vi "frequency_sweep_agilent.vi"() -> ()   [LabVIEW 2017]
uses:
  controls/State.ctl
  controls/Data.ctl
  field_sweep_Agilent/Controls/Instruments.ctl
  <vilib>/Utility/error.llb/DialogType.ctl
  <vilib>/DAQmx/write.llb/DAQmx Write (Analog DBL 1Chan 1Samp).vi
  <vilib>/DAQmx/create/channels.llb/DAQmx Create Channel (AO-Voltage-Basic).vi
  <vilib>/DAQmx/miscellaneous.llb/DAQmx Fill In Error Info.vi
  <instrlib>/Keysight PNA Series/Keysight PNA Series.lvlib
panel:
  in  "Average Mode":i32(ring) items=["Point", "Sweep"]
  out "Field, Oe":dbl=17.9778 format="%#_4f"
  in  "IF Bandwidth":dbl(ring)=300.0 items=["10 Hz"=10.0, "30 Hz"=30.0, "100 Hz"=100.0, "300 Hz"=300.0, "1 KHz"=1000.0, "3 KHz"=3000.0, "10 KHz"=10000.0, "30 KHz"=30000.0]
  in  "Sweep Generation":i32(ring)=1 items=["Stepped", "Analog"]
  in  "Source Port":i32=1
  in  "Display Format":i32(ring) items=["Magnitude Linear", "Magnitude Logarithmic", "Phase", "Unwrapped phase", "Imaginary", "Real", "Polar", "Smith Chart", "Smith Admittance", "SWR", "Group Delay", "Kelvin", "Fahrenheit", "Celsius"]
  in  "S-parameter":i32(ring) items=["S11", "S12", "S21", "S22"]
  in  "Temp. Contr. Name (in)":refnum<visa-resource-name>="LakeShore336"
  in  "VNA name (in)":refnum<visa-resource-name>="vna"
  in  "Gaussmeter Name (in)":refnum<visa-resource-name>="Lakeshore_475"
  in  "DAQ channel (in)":tag="DAQ_6363/ao1"
  in  "Reference H Field On/Off":bool
  in  "Averaging Points":i32=1 min=1 max=3201 step=1
  in  "Exit Button":bool
  in  "Reference H Field (Oe)":dbl=4400.0 min=-4400.0 max=4400.0
  in  "H Field (Oe)":dbl=1000.0 min=-6000.0 max=6000.0
  in  "Save Button":bool
  out "Status":string="Off"
  out "Cursor":cluster{"x":dbl, "y":dbl} {"x" format="%.2f"; "y" format="%.5f"}
  out "Error Out":errorcluster={"status"=FALSE, "code"=1073676293, "source"="VISA Read in Keysight PNA Series.lvlib:Error Query.vi->Keysight PNA Series.lvlib:Close.vi->frequency_sweep_agilent.vi"}
  in  "Error In (no error)":errorcluster
  out "SpectrumGraph":cluster{"Field":dbl[], "Signal":dbl[]}(graph)
  in  "Start Button":bool
  in  "Stop Button":bool
  in  "Output Power (dBm)":dbl min=-25.0 max=50.0 step=0.5
  in  "Number of Points":i32=1000 min=1 max=3201 step=1
  in  "Stop frequency (GHz)":dbl=6.0 caption="Stop H Field (Oe)" min=0.01 max=26.5 format="%#_6f"
  in  "Start frequency (GHz)":dbl=1.0 min=0.01 max=26.5 format="%#_6f"
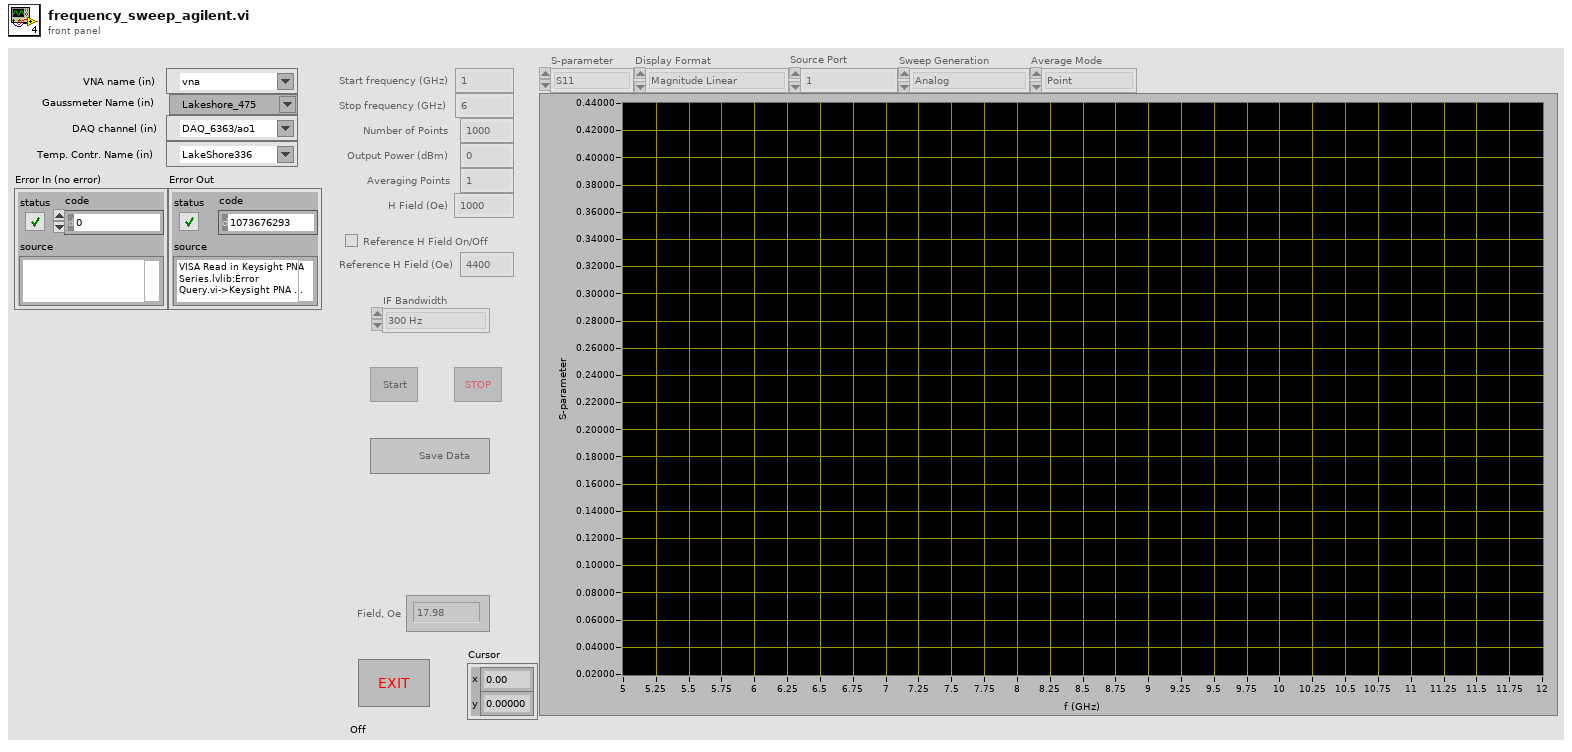
[diagram p1: front panel]
types:
  T1 = typedef "Instruments.ctl" = cluster{"Gaussmeter Name":refnum<visa-resource-name>, "VNA name":refnum<visa-resource-name>, "DAQ channel":tag, "DAQ task":refnum<k21>, "Temp. Contr. Name":refnum<visa-resource-name>}
  T2 = typedef "Data.ctl" = cluster{"Frequency":dbl[], "Signal":dbl[], "Ref signal":dbl[]}
  T3 = typedef "State.ctl" = enum16{"Init", "Idle", "Configuring", "Sweeping to ref", "Measuring ref", "Sweeping to H", "Measuring H", "Sweeping down", "Shutdown"}
  T4 = typedef "DialogType.ctl" = u16
  T5 = typedef "LVPoint32TypeDef.ctl" = cluster{"Horizontal":i32, "Vertical":i32}
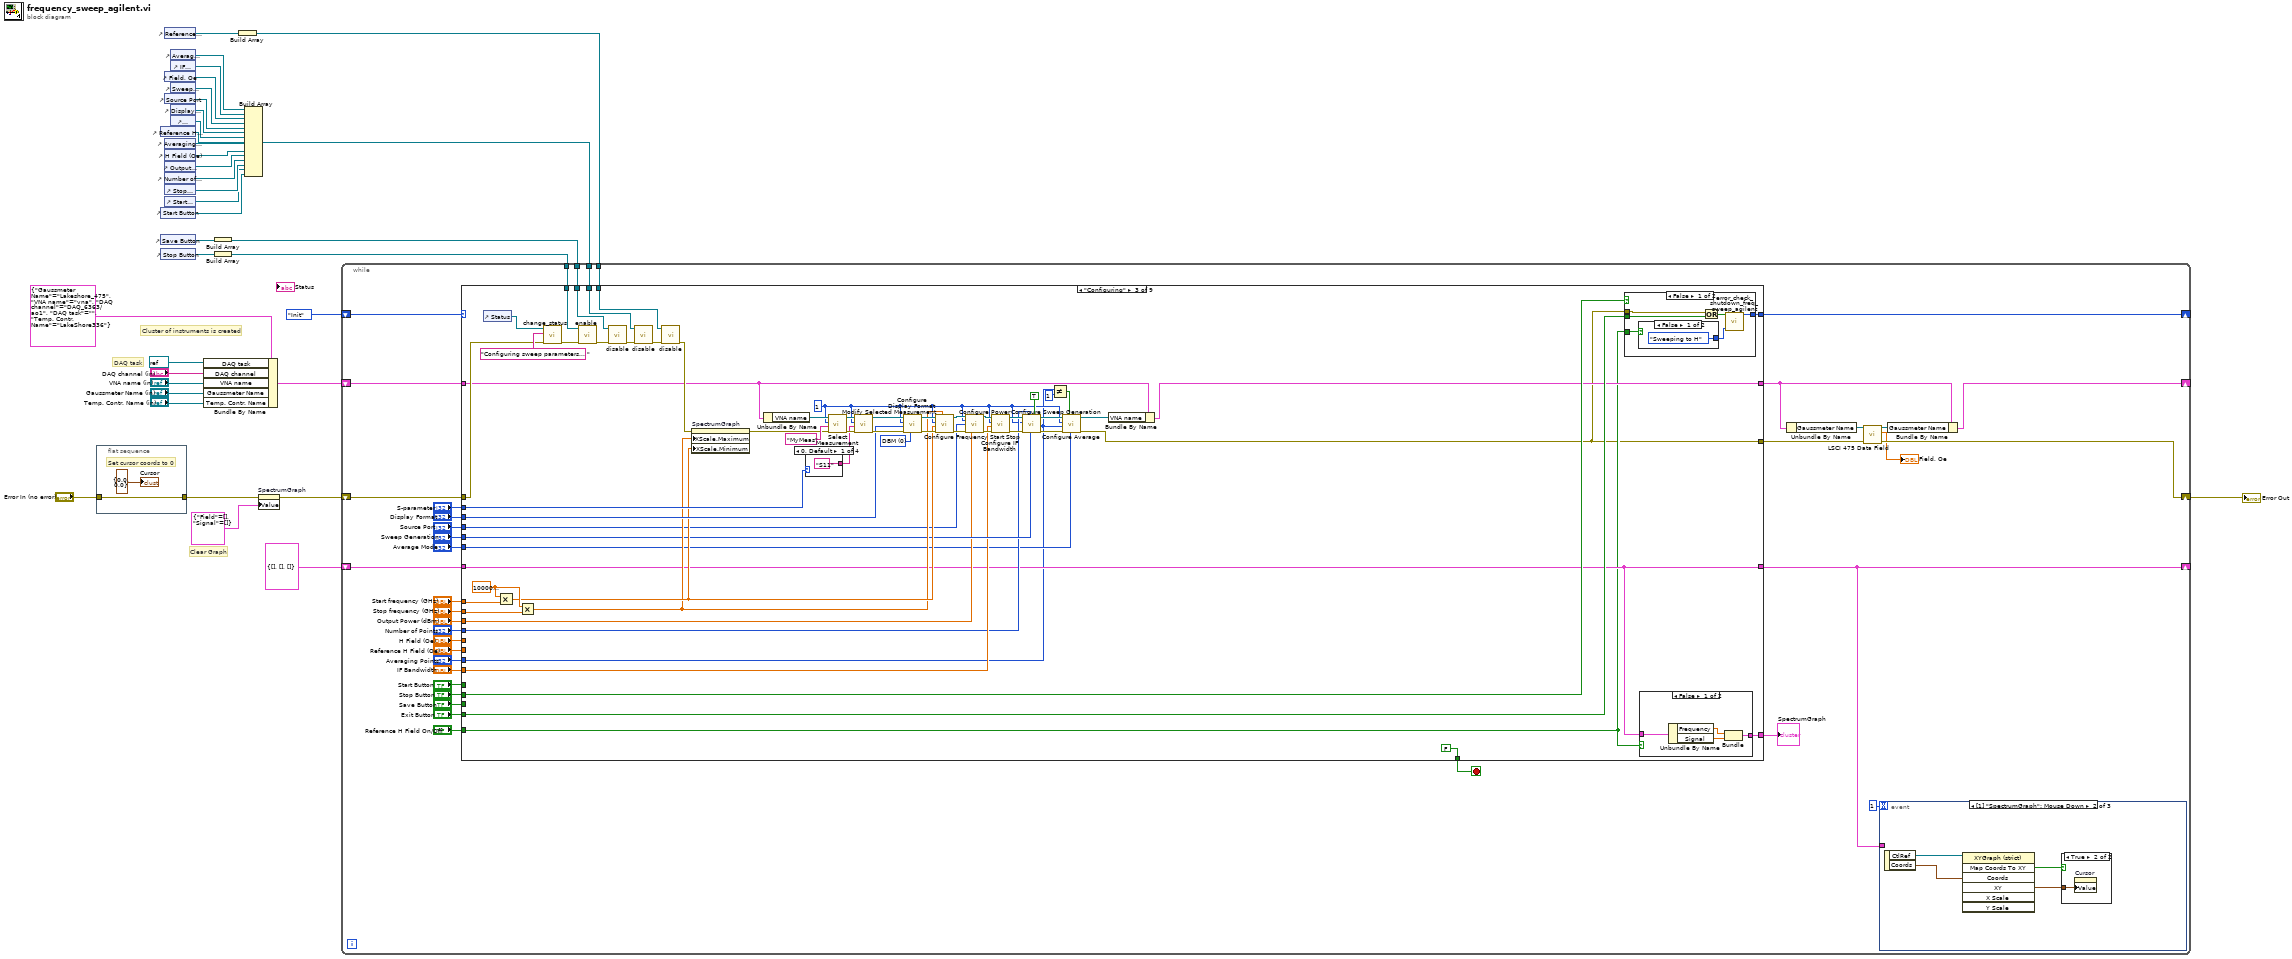
[diagram p0: block diagram]
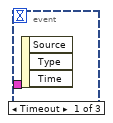
[diagram p2: hidden frame]
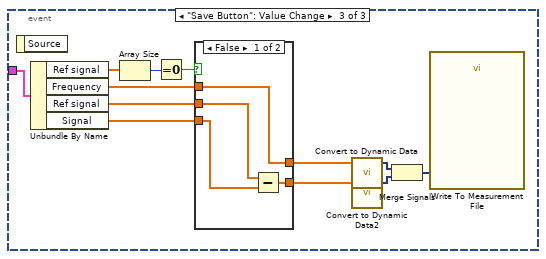
[diagram p4: hidden frame]
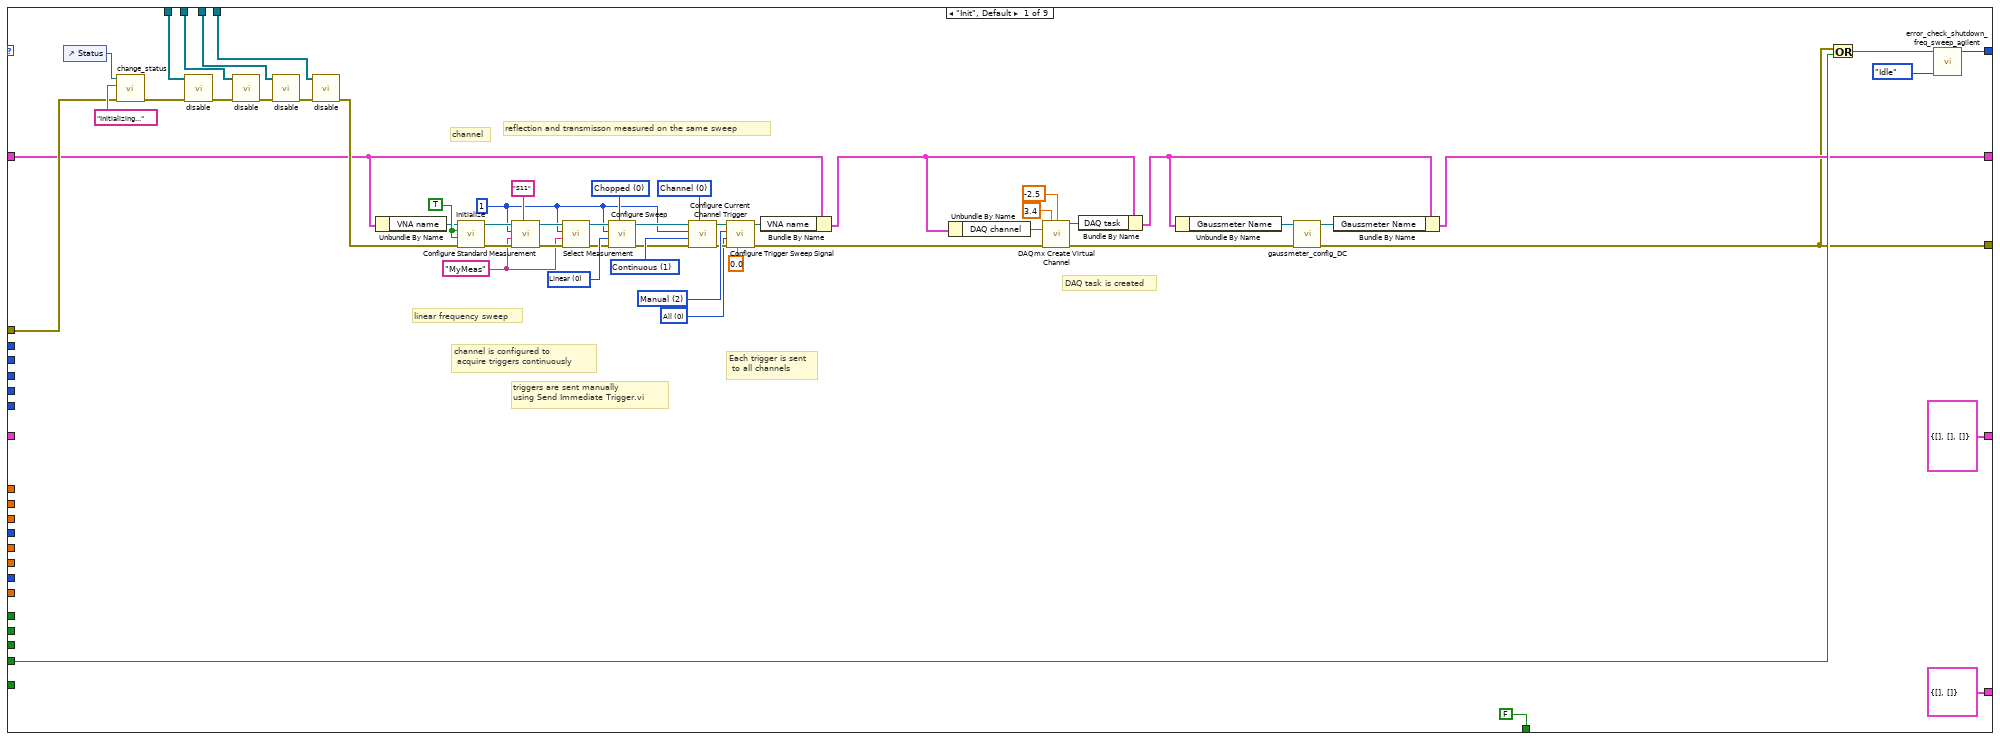
[diagram p6: hidden frame]
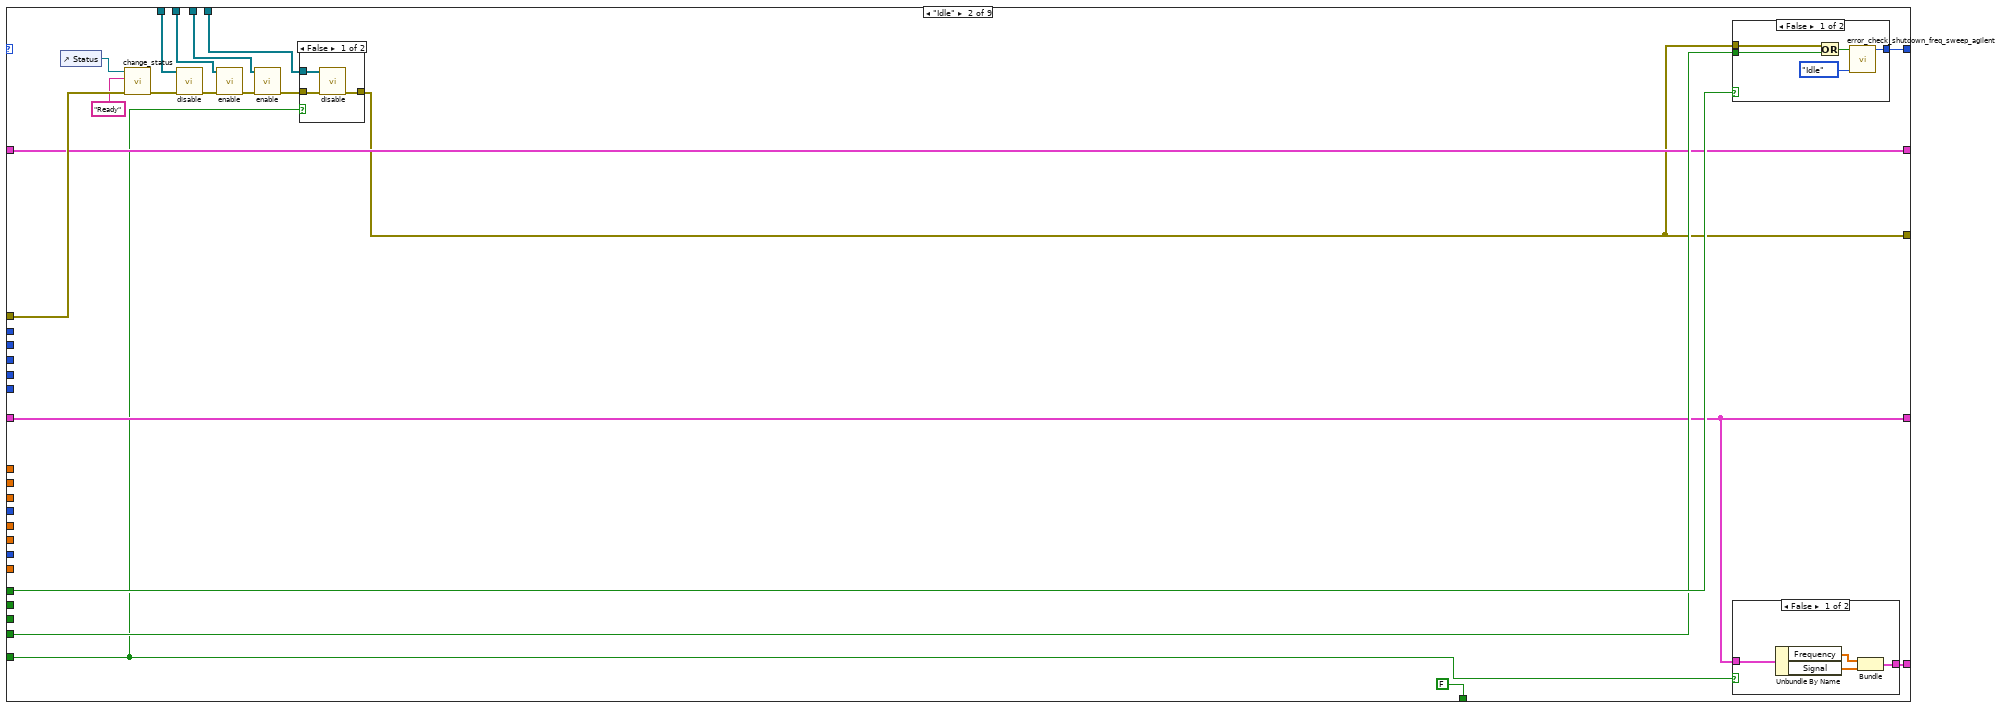
[diagram p7: hidden frame]
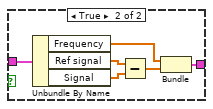
[diagram p8: hidden frame]
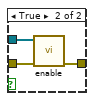
[diagram p9: hidden frame]
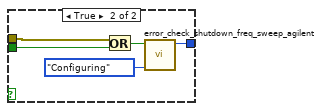
[diagram p10: hidden frame]
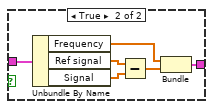
[diagram p11: hidden frame]
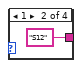
[diagram p12: hidden frame]
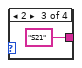
[diagram p13: hidden frame]
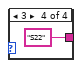
[diagram p14: hidden frame]
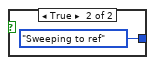
[diagram p15: hidden frame]
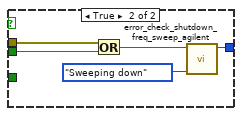
[diagram p16: hidden frame]
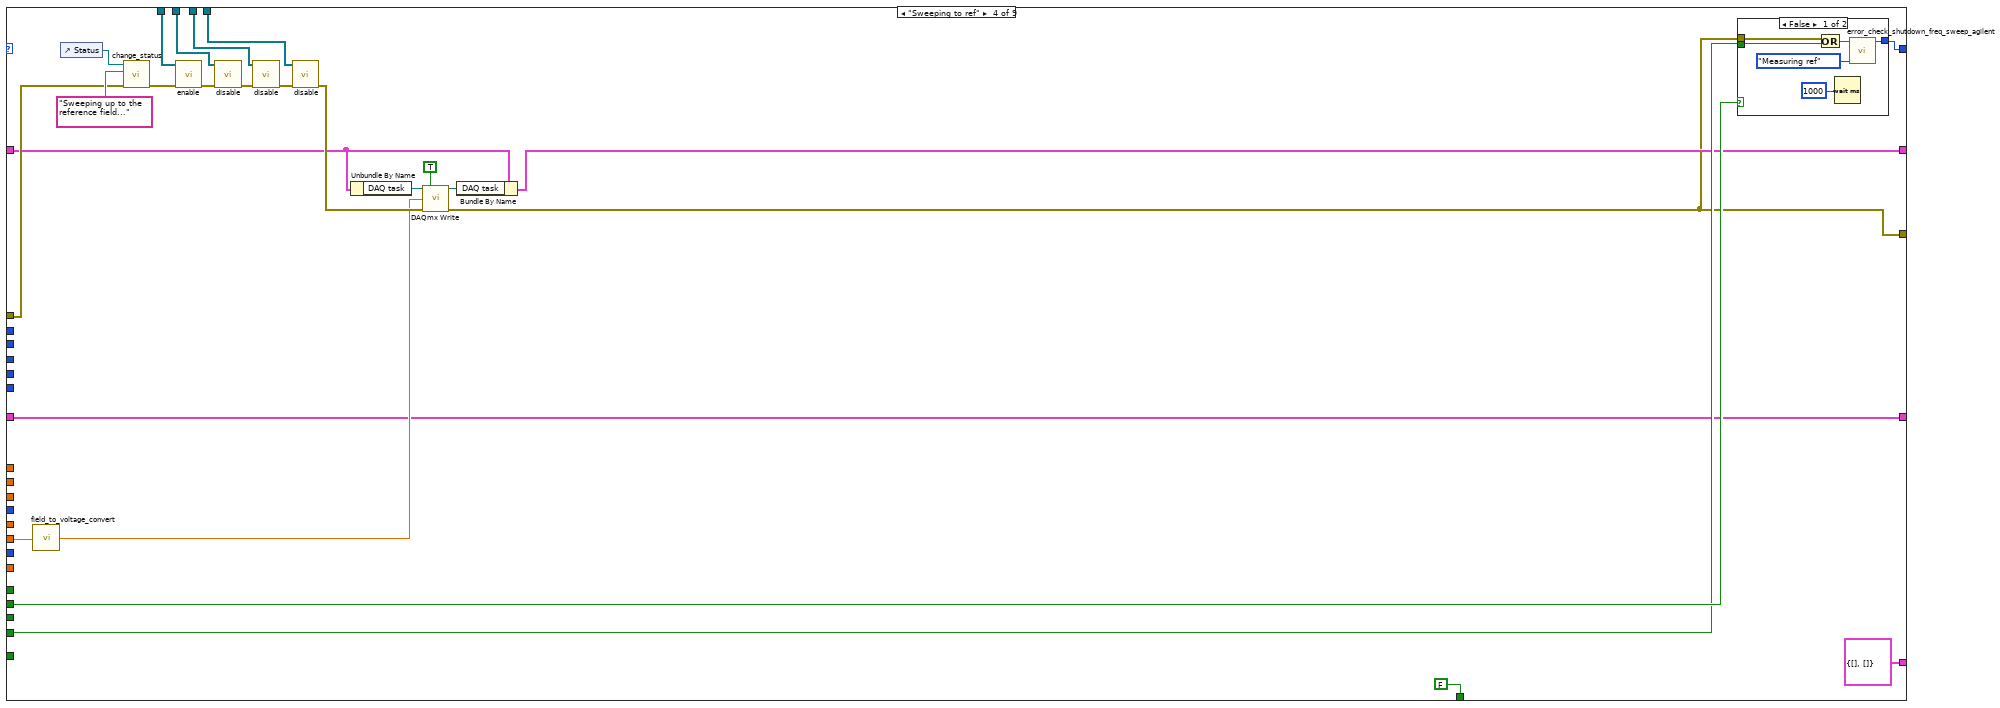
[diagram p17: hidden frame]
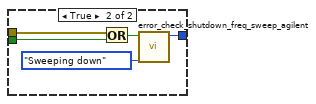
[diagram p18: hidden frame]
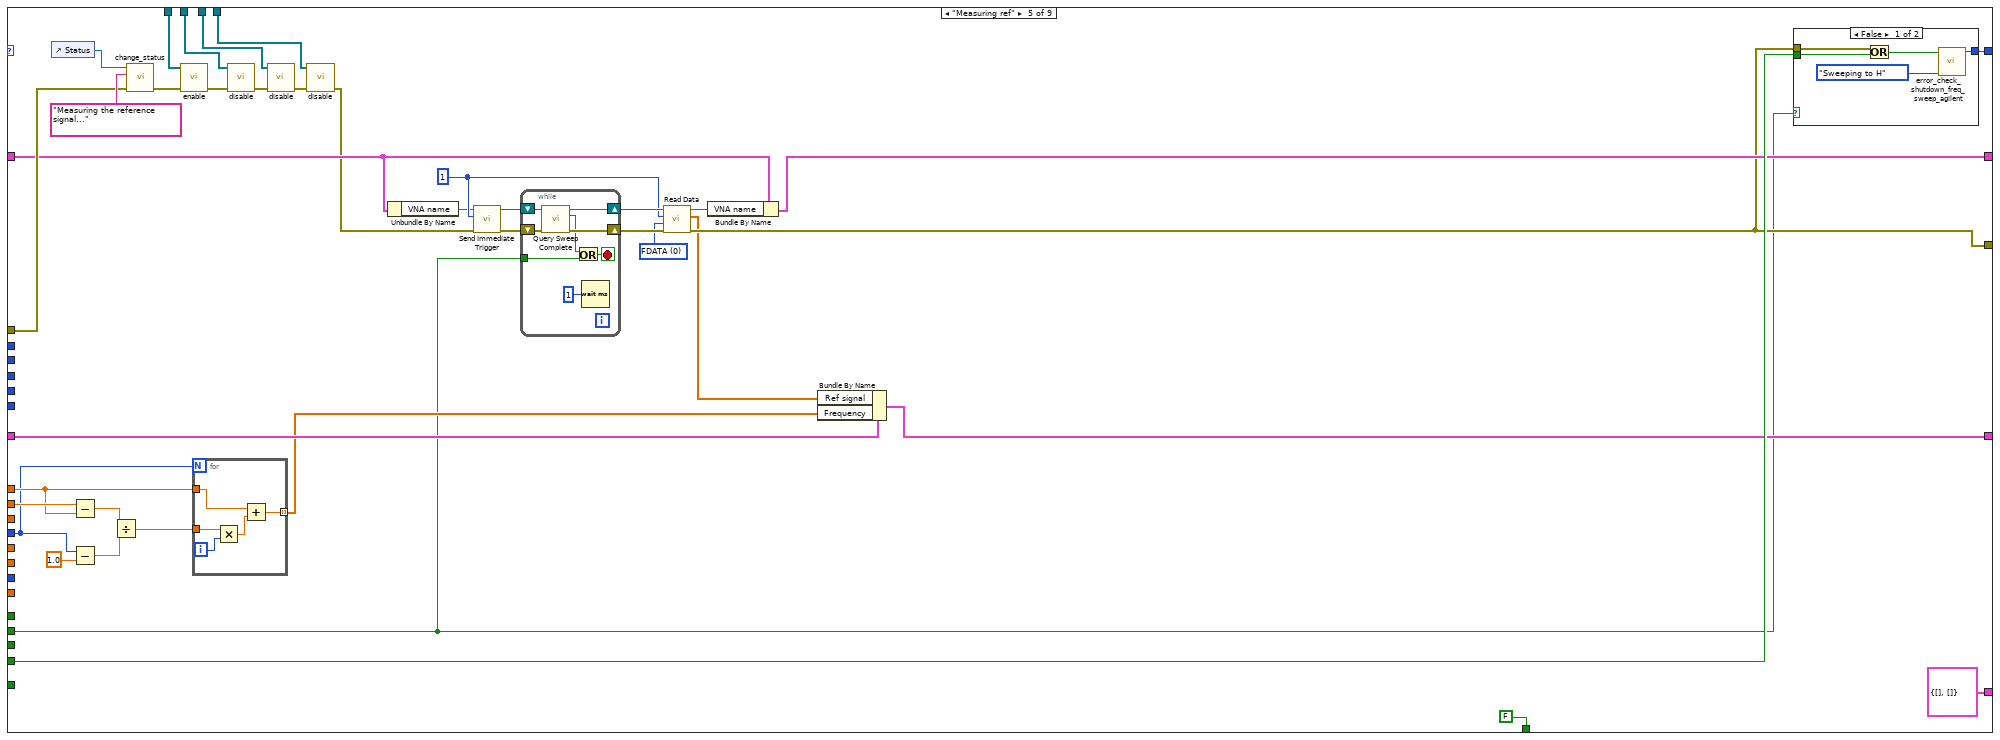
[diagram p19: hidden frame]
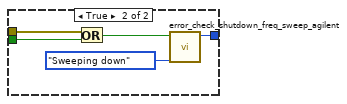
[diagram p20: hidden frame]
diagram:
  # "Cluster of instruments is created"
  # "DAQ task"
  # "Clear Graph"
  n1 = flat-sequence {
    tunnel: "Error In (no error)" -> [w38]
    tunnel: [w38] -> w9
    frame #0 {
      # "Set cursor coords to 0"
      "Cursor" <- cluster{"x":dbl, "y":dbl} {"x"=0.0, "y"=0.0} ("Cursor")
    }
  }
  n2 = control-ref of="Reference H Field On/Off"() -> (w8:refnum<vi>)
  n3 = control-ref of="Start Button"() -> (w18:refnum<vi>)
  n4 = control-ref of="Save Button"() -> (w28:refnum<vi>)
  n5 = control-ref of="Stop Button"() -> (w31:refnum<vi>)
  n6 = control-ref of="Reference H Field (Oe)"() -> (w20:refnum<vi>)
  n7 = control-ref of="Field, Oe"() -> (w3:refnum<vi>)
  n8 = control-ref of="Source Port"() -> (w5:refnum<vi>)
  n9 = control-ref of="Averaging Points"() -> (w26:refnum<vi>)
  n10 = control-ref of="H Field (Oe)"() -> (w36:refnum<vi>)
  n11 = control-ref of="Output Power (dBm)"() -> (w35:refnum<vi>)
  n12 = control-ref of="Number of Points"() -> (w34:refnum<vi>)
  n13 = control-ref of="Stop frequency (GHz)"() -> (w33:refnum<vi>)
  n14 = control-ref of="Start frequency (GHz)"() -> (w32:refnum<vi>)
  n15 = control-ref of="Average Mode"() -> (w1:refnum<vi>)
  n16 = control-ref of="IF Bandwidth"() -> (w2:refnum<vi>)
  n17 = control-ref of="Sweep Generation"() -> (w4:refnum<vi>)
  n18 = control-ref of="Display Format"() -> (w6:refnum<vi>)
  n19 = control-ref of="S-parameter"() -> (w7:refnum<vi>)
  n20 = Bundle By Name(cluster=T1 {"Gaussmeter Name"="Lakeshore_475", "VNA name"="vna", "DAQ channel"="DAQ_6363/ao1", "DAQ task"="", "Temp. Contr. Name"="LakeShore336"} ("Cluster"), "DAQ task"=refnum<k21> refnum ("task in"), "DAQ channel"="DAQ channel (in)", "VNA name"="VNA name (in)", "Gaussmeter Name"="Gaussmeter Name (in)", "Temp. Contr. Name"="Temp. Contr. Name (in)") -> (w11:T1)
  n21 = Build Array(w28) -> (w27:refnum<vi>[])
  n22 = Build Array(w31) -> (w29:refnum<vi>[])
  n23 = Build Array(w20) -> (w19:refnum<vi>[])
  n24 = Build Array(w1, w2, w3, w4, w5, w6, w7, w8, w26, w36, w35, w34, w33, w32, w18) -> (w30:refnum<vi>[])
  n25 = property on="SpectrumGraph" class="XYGraph (strict)"(error in=w9, "Value"=cluster{"Field":dbl[], "Signal":dbl[]} {"Field"=[], "Signal"=[]} ("SpectrumGraph")) -> (error out=w24:errorcluster)  [unwired: 1 in, 1 out]
  n26 = while {
    shift-right: [w57] -> _
    shift-left: State."Init" -> [w58]
    tunnel: w30 -> [w76]
    tunnel: w29 -> [w75]
    shift-right: [w44] -> w25
    shift-left: w24 -> [w74]
    tunnel: w27 -> [w73]
    shift-right: [w47] -> _
    shift-left: T2 {"Frequency"=[], "Signal"=[], "Ref signal"=[]} -> [w59]
    tunnel: w19 -> [w55]
    shift-right: [w41] -> _
    shift-left: w11 -> [w54]
    stop <- w68 stop-if-true
    n27 = case shown="\"Configuring\"" w58 {
      tunnel: w76 -> [w148 w172 w256 w308 w361 w408 w471 w527 w573]
      tunnel: w75 -> [w154 w174 w255 w310 w363 w411 w473 w525 w575]
      tunnel: w74 -> [w150 w169 w253 w306 w356 w406 w470 w528 w571]
      tunnel: [w145 w163 w248 w304 w354 w401 w450 w522 State."Shutdown" ("Enum")] -> w57
      tunnel: [w102 w158 w206 w290 w338 w390 w449 w503 w560] -> w46
      tunnel: w73 -> [w149 w173 w257 w309 w362 w409 w472 w526 w574]
      tunnel: "Start Button" -> [_ w166 _ _ _ _ _ _ _]
      tunnel: "Stop Button" -> [_ _ w250 w305 w325 w403 w435 _ _]
      tunnel: "Save Button" -> [_ _ _ _ _ _ _ _ _]
      tunnel: "Exit Button" -> [w146 w165 w249 w303 w355 w402 w468 w523 _]
      tunnel: [FALSE FALSE FALSE FALSE FALSE FALSE FALSE FALSE TRUE] -> w68
      tunnel: "Start frequency (GHz)" -> [_ _ w252 _ w332 _ w441 _ _]
      tunnel: "Stop frequency (GHz)" -> [_ _ w251 _ w333 _ w446 _ _]
      tunnel: "Output Power (dBm)" -> [_ _ w217 _ _ _ _ _ _]
      tunnel: "Number of Points" -> [_ _ w213 _ w331 _ w442 _ _]
      tunnel: "H Field (Oe)" -> [_ _ _ _ _ w404 _ _ _]
      tunnel: "Reference H Field (Oe)" -> [_ _ _ w301 _ _ _ _ _]
      tunnel: "Averaging Points" -> [_ _ w202 _ _ _ _ _ _]
      tunnel: w59 -> [_ w156 w211 w289 w330 w388 w448 w501 _]
      tunnel: [T2 {"Frequency"=[], "Signal"=[], "Ref signal"=[]} w156 w211 w289 w327 w388 w437 w501 T2 {"Frequency"=[], "Signal"=[], "Ref signal"=[]}] -> w47
      tunnel: "S-parameter" -> [_ _ w227 _ _ _ _ _ _]
      tunnel: "Reference H Field On/Off" -> [_ w155 w210 _ _ w387 w438 w500 _]
      tunnel: w55 -> [w139 w160 w244 w298 w350 w398 w465 w516 w565]
      tunnel: w54 -> [w114 w159 w215 w293 w341 w393 w454 w506 w544]
      tunnel: [w105 w159 w214 w292 w340 w392 w453 w504 w544] -> w42
      tunnel: "Display Format" -> [_ _ w226 _ _ _ _ _ _]
      tunnel: "Source Port" -> [_ _ w219 _ _ _ _ _ _]
      tunnel: "Sweep Generation" -> [_ _ w218 _ _ _ _ _ _]
      tunnel: "IF Bandwidth" -> [_ _ w216 _ _ _ _ _ _]
      tunnel: [cluster{"Frequency":dbl[], "Signal":dbl[]} {"Frequency"=[], "Signal"=[]} w157 w212 cluster{"Frequency":dbl[], "Signal":dbl[]} {"Frequency"=[], "Signal"=[]} cluster{"Frequency":dbl[], "Signal":dbl[]} {"Frequency"=[], "Signal"=[]} w389 w436 w502 cluster{"Frequency":dbl[], "Signal":dbl[]} {"Frequency"=[], "Signal"=[]}] -> w48
      tunnel: "Average Mode" -> [_ _ w205 _ _ _ _ _ _]
      frame "Init", Default {
        w121 = 0 items=["All", "Current"] ("Trigger Scope (0: All)")
        w122 = 0 items=["Channel", "Sweep", "Point", "Trace"] ("Trigger Mode (0: Channel)")
        w125 = 1 items=["Hold", "Continuous", "Groups", "Single"] ("Trigger Condition (1: Continuous)")
        w126 = 2 items=["Immediate", "External", "Manual"] ("Trigger Source (0: Immediate)")
        w132 = 0 items=["Chopped", "Alternate"] ("Sweep Mode (0: Chopped)")
        w133 = 0 items=["Linear", "Logarithmic", "Power", "CW", "Segment", "Phase"] ("Sweep Type (0: Linear)")
        w127 = "MyMeas" ("Measurement Name (CH1_S11_1)")
        w116 = 1 ("Channel (1)")
        w138 = TRUE ("ID Query (True)")
        # "DAQ task is created"
        # "channel"
        # "reflection and transmisson measured on the same sweep"
        # "Each trigger is sent\n to all channels"
        # "triggers are sent manually\nusing Send Immediate Trigger.vi"
        # "channel is configured to\n acquire triggers continuously"
        # "linear frequency sweep"
        n28 = control-ref of="Status"() -> (w152:refnum<vi>)
        n29 = call "change_status.vi"("error in (no error)"=w150, "String"="Initializing...", "String in"=w152) -> ("error out"=w153:errorcluster)  [unwired: 8 in]
        n30 = call "disable.vi"("error in (no error)"=w153, "Array"=w154) -> ("error out"=w141:errorcluster)  [unwired: 9 in]
        n31 = call "disable.vi"("error in (no error)"=w141, "Array"=w149) -> ("error out"=w147:errorcluster)  [unwired: 9 in]
        n32 = call "disable.vi"("error in (no error)"=w147, "Array"=w148) -> ("error out"=w140:errorcluster)  [unwired: 9 in]
        n33 = call "disable.vi"("error in (no error)"=w140, "Array"=w139) -> ("error out"=w115:errorcluster)  [unwired: 9 in]
        n34 = Unbundle By Name(w114) -> ("VNA name"=w134:refnum<visa-resource-name>)
        n35 = call <instrlib>:"Initialize.vi"("error in (no error)"=w115, "Reset (True)"=w138, "ID Query (True)"=w138, "VISA resource name"=w134) -> ("error out"=w137:errorcluster, "VISA resource name out"=w136:refnum<visa-resource-name>)  [unwired: 6 in]
        n36 = call <instrlib>:"Configure Standard Measurement.vi"("Measurement Parameters (S11)"="S11", "error in (no error)"=w137, "Measurement Name (CH1_S11_1)"=w127, "Channel (1)"=w116, "VISA resource name"=w136) -> ("error out"=w130:errorcluster, "VISA resource name out"=w131:refnum<visa-resource-name>)  [unwired: 5 in]
        n37 = call <instrlib>:"Select Measurement.vi"("error in (no error)"=w130, "Measurement Name (CH1_S11_1)"=w127, "Channel (1)"=w116, "VISA resource name"=w131) -> ("error out"=w128:errorcluster, "VISA resource name out"=w129:refnum<visa-resource-name>)  [unwired: 6 in]
        n38 = call <instrlib>:"Configure Sweep.vi"("Sweep Mode (0: Chopped)"=w132, "error in (no error)"=w128, "Sweep Type (0: Linear)"=w133, "Channel (1)"=w116, "VISA resource name"=w129) -> ("error out"=w119:errorcluster, "VISA resource name out"=w118:refnum<visa-resource-name>)  [unwired: 5 in]
        n39 = call <instrlib>:"Configure Current Channel Trigger.vi"("Trigger Mode (0: Channel)"=w122, "error in (no error)"=w119, "Trigger Condition (1: Continuous)"=w125, "Channel (1)"=w116, "VISA resource name"=w118) -> ("error out"=w124:errorcluster, "VISA resource name out"=w123:refnum<visa-resource-name>)  [unwired: 5 in]
        n40 = call <instrlib>:"Configure Trigger Sweep Signal.vi"("Delay (0 s)"=0.0, "error in (no error)"=w124, "Trigger Scope (0: All)"=w121, "Trigger Source (0: Immediate)"=w126, "VISA resource name"=w123) -> ("error out"=w107:errorcluster, "VISA resource name out"=w117:refnum<visa-resource-name>)  [unwired: 5 in]
        n41 = Bundle By Name(cluster=w114, "VNA name"=w117) -> (w104:T1)
        n42 = Unbundle By Name(w104) -> ("DAQ channel"=w111:tag)
        n43 = call-poly <vilib>:"DAQmx Create Virtual Channel.vi"("maximum value"=3.4, "minimum value"=-2.5, "physical channels"=w111, "error in"=w107) -> ("task out"=w110:refnum<k21>, "error out"=w109:errorcluster)  [unwired: 10 in]
        n44 = Bundle By Name(cluster=w104, "DAQ task"=w110) -> (w103:T1)
        n45 = Unbundle By Name(w103) -> ("Gaussmeter Name"=w106:refnum<visa-resource-name>)
        n46 = call "gaussmeter_config_DC.vi"("error in (no error)"=w109, "VISA Refnum in"=w106) -> ("error out"=w102:errorcluster, "VISA Refnum out"=w108:refnum<visa-resource-name>)  [unwired: 8 in]
        n47 = Bundle By Name(cluster=w103, "Gaussmeter Name"=w108) -> (w105:T1)
        n48 = Or(x=w102, y=w146) -> (x .or. y?=w144:bool)
        n49 = call "error_check_shutdown_freq_sweep_agilent.vi"(8:State."Idle", "Boolean"=w144) -> (3:w145:T3)  [unwired: 9 in]
      }
      frame "Idle" {
        n50 = control-ref of="Status"() -> (w168:refnum<vi>)
        n51 = call "change_status.vi"("error in (no error)"=w169, "String"="Ready", "String in"=w168) -> ("error out"=w170:errorcluster)  [unwired: 8 in]
        n52 = call "disable.vi"("error in (no error)"=w170, "Array"=w174) -> ("error out"=w162:errorcluster)  [unwired: 9 in]
        n53 = call "enable.vi"("error in (no error)"=w162, "Array"=w173) -> ("error out"=w171:errorcluster)  [unwired: 9 in]
        n54 = call "enable.vi"("error in (no error)"=w171, "Array"=w172) -> ("error out"=w161:errorcluster)  [unwired: 9 in]
        n55 = case shown="False" w155 {
          tunnel: w161 -> [w187 w190]
          tunnel: [w185 w189] -> w158
          tunnel: w160 -> [w186 w188]
          frame False {
            n56 = call "disable.vi"("error in (no error)"=w187, "Array"=w186) -> ("error out"=w185:errorcluster)  [unwired: 9 in]
          }
          frame True {
            n57 = call "enable.vi"("error in (no error)"=w190, "Array"=w188) -> ("error out"=w189:errorcluster)  [unwired: 9 in]
          }
        }
        n58 = case shown="False" w166 {
          tunnel: [w192 w198] -> w163
          tunnel: w165 -> [w195 w200]
          tunnel: w158 -> [w191 w196]
          frame False {
            n59 = Or(x=w191, y=w195) -> (x .or. y?=w194:bool)
            n60 = call "error_check_shutdown_freq_sweep_agilent.vi"(8:State."Idle", "Boolean"=w194) -> (3:w192:T3)  [unwired: 9 in]
          }
          frame True {
            n61 = Or(x=w196, y=w200) -> (x .or. y?=w199:bool)
            n62 = call "error_check_shutdown_freq_sweep_agilent.vi"(8:State."Configuring", "Boolean"=w199) -> (3:w198:T3)  [unwired: 9 in]
          }
        }
        n63 = case shown="False" w155 {
          tunnel: w156 -> [w178 w184]
          tunnel: [w175 w179] -> w157
          frame False {
            n64 = Unbundle By Name(w178) -> ("Frequency"=w177:dbl[], "Signal"=w176:dbl[])
            n65 = Bundle("Frequency"=w177, "Signal"=w176) -> (w175:cluster{"Frequency":dbl[], "Signal":dbl[]})  [unwired: 1 in]
          }
          frame True {
            n66 = Unbundle By Name(w184) -> ("Frequency"=w181:dbl[], "Ref signal"=w183:dbl[], "Signal"=w182:dbl[])
            n67 = Subtract(x=w183, y=w182) -> (x-y=w180:dbl[])
            n68 = Bundle("Frequency"=w181, w180) -> (w179:cluster{"Frequency":dbl[], dbl[]})  [unwired: 1 in]
          }
        }
      }
      frame "Configuring" {
        w229 = 0 items=["DBM", "DBMV", "DBMA", "W", "V", "A"] ("Unit (0: DBM)")
        w204 = 1 ("Channel (1)")
        w242 = 1000000000.0 ("x")
        n69 = control-ref of="Status"() -> (w254:refnum<vi>)
        n70 = Multiply(x=w242, y=w252) -> (x*y=w221:dbl)
        n71 = Multiply(x=w242, y=w251) -> (x*y=w220:dbl)
        n72 = call "change_status.vi"("error in (no error)"=w253, "String"="Configuring sweep parameters... ", "String in"=w254) -> ("error out"=w259:errorcluster)  [unwired: 8 in]
        n73 = call "enable.vi"("error in (no error)"=w259, "Array"=w255) -> ("error out"=w246:errorcluster)  [unwired: 9 in]
        n74 = call "disable.vi"("error in (no error)"=w246, "Array"=w257) -> ("error out"=w260:errorcluster)  [unwired: 9 in]
        n75 = call "disable.vi"("error in (no error)"=w260, "Array"=w256) -> ("error out"=w245:errorcluster)  [unwired: 9 in]
        n76 = call "disable.vi"("error in (no error)"=w245, "Array"=w244) -> ("error out"=w243:errorcluster)  [unwired: 9 in]
        n77 = property on="SpectrumGraph" class="XYGraph (strict)"(error in=w243, "XScale.Maximum"=w220, "XScale.Minimum"=w221) -> (error out=w228:errorcluster)  [unwired: 1 in, 1 out]
        n78 = Unbundle By Name(w215) -> ("VNA name"=w236:refnum<visa-resource-name>)
        n79 = case shown="0, Default" w227 {
          tunnel: ["S11" ("Measurement Parameters (S11)") "S12" ("Measurement Parameters (S11)") "S21" ("Measurement Parameters (S11)") "S22" ("Measurement Parameters (S11)")] -> w230
          frame 0, Default {
          }
          frame 1 {
          }
          frame 2 {
          }
          frame 3 {
          }
        }
        n80 = call <instrlib>:"Select Measurement.vi"("error in (no error)"=w228, "Measurement Name (CH1_S11_1)"="MyMeas", "Channel (1)"=w204, "VISA resource name"=w236) -> ("error out"=w233:errorcluster, "VISA resource name out"=w234:refnum<visa-resource-name>)  [unwired: 6 in]
        n81 = call <instrlib>:"Modify Selected Measurement.vi"("error in (no error)"=w233, "Measurement Parameter (S11)"=w230, "Channel (1)"=w204, "VISA resource name"=w234) -> ("error out"=w231:errorcluster, "VISA resource name out"=w232:refnum<visa-resource-name>)  [unwired: 6 in]
        n82 = call <instrlib>:"Configure Display Format.vi"("Unit (0: DBM)"=w229, "error in (no error)"=w231, "Display Format (0: Magnitude Linear)"=w226, "Channel (1)"=w204, "VISA resource name"=w232) -> ("error out"=w224:errorcluster, "VISA resource name out"=w225:refnum<visa-resource-name>)  [unwired: 5 in]
        n83 = call <instrlib>:"Configure Frequency Start Stop.vi"("Stop Frequency (2E+6 Hz)"=w220, "error in (no error)"=w224, "Start Frequency (1E+6 Hz)"=w221, "Channel (1)"=w204, "VISA resource name"=w225) -> ("error out"=w222:errorcluster, "VISA resource name out"=w223:refnum<visa-resource-name>)  [unwired: 5 in]
        n84 = call <instrlib>:"Configure Power.vi"("VISA resource name"=w223, "Channel (1)"=w204, "Port (1)"=w219, "error in (no error)"=w222, "Power Level (0 dBm)"=w217) -> ("VISA resource name out"=w240:refnum<visa-resource-name>, "error out"=w241:errorcluster)  [unwired: 9 in]
        n85 = call <instrlib>:"Configure IF Bandwidth.vi"("error in (no error)"=w241, "Bandwidth (100000 Hz)"=w216, "Channel (1)"=w204, "VISA resource name"=w240) -> ("error out"=w238:errorcluster, "VISA resource name out"=w239:refnum<visa-resource-name>)  [unwired: 6 in]
        n86 = call <instrlib>:"Configure Sweep Generation.vi"("Auto Sweep or Dwell Time (T: Enable)"=TRUE, "Sweep Generation (1: Analog)"=w218, "Sweep Points (201)"=w213, "error in (no error)"=w238, "Channel (1)"=w204, "VISA resource name"=w239) -> ("error out"=w208:errorcluster, "VISA resource name out"=w209:refnum<visa-resource-name>)  [unwired: 4 in]
        n87 = Not Equal?(x=w202, y=1) -> (x != y?=w201:bool)
        n88 = call <instrlib>:"Configure Average.vi"("Average Mode (1: Sweep)"=w205, "Enable Average (F: Disable)"=w201, "error in (no error)"=w208, "Average Count (1)"=w202, "Channel (1)"=w204, "VISA resource name"=w209) -> ("error out"=w206:errorcluster, "VISA resource name out"=w207:refnum<visa-resource-name>)  [unwired: 4 in]
        n89 = Bundle By Name(cluster=w215, "VNA name"=w207) -> (w214:T1)
        n90 = case shown="False" w250 {
          tunnel: [w277 w285] -> w248
          tunnel: w249 -> [w280 w287]
          tunnel: w210 -> [w276 _]
          tunnel: w206 -> [w275 w283]
          frame False {
            n91 = case shown="False" w276 {
              tunnel: [State."Sweeping to H" State."Sweeping to ref"] -> w278
              frame False {
              }
              frame True {
              }
            }
            n92 = Or(x=w275, y=w280) -> (x .or. y?=w279:bool)
            n93 = call "error_check_shutdown_freq_sweep_agilent.vi"(8:w278, "Boolean"=w279) -> (3:w277:T3)  [unwired: 9 in]
          }
          frame True {
            n94 = Or(x=w283, y=w287) -> (x .or. y?=w286:bool)
            n95 = call "error_check_shutdown_freq_sweep_agilent.vi"(8:State."Sweeping down", "Boolean"=w286) -> (3:w285:T3)  [unwired: 9 in]
          }
        }
        n96 = case shown="False" w210 {
          tunnel: w211 -> [w264 w270]
          tunnel: [w261 w265] -> w212
          frame False {
            n97 = Unbundle By Name(w264) -> ("Frequency"=w263:dbl[], "Signal"=w262:dbl[])
            n98 = Bundle("Frequency"=w263, "Signal"=w262) -> (w261:cluster{"Frequency":dbl[], "Signal":dbl[]})  [unwired: 1 in]
          }
          frame True {
            n99 = Unbundle By Name(w270) -> ("Frequency"=w267:dbl[], "Ref signal"=w269:dbl[], "Signal"=w268:dbl[])
            n100 = Subtract(x=w269, y=w268) -> (x-y=w266:dbl[])
            n101 = Bundle("Frequency"=w267, w266) -> (w265:cluster{"Frequency":dbl[], dbl[]})  [unwired: 1 in]
          }
        }
      }
      frame "Sweeping to ref" {
        n102 = call "field_to_voltage_convert.vi"("Start H Field (Oe)"=w301) -> ("Numeric"=w291:dbl)
        n103 = control-ref of="Status"() -> (w307:refnum<vi>)
        n104 = call "change_status.vi"("error in (no error)"=w306, "String"="Sweeping up to the reference field...", "String in"=w307) -> ("error out"=w312:errorcluster)  [unwired: 8 in]
        n105 = call "enable.vi"("error in (no error)"=w312, "Array"=w310) -> ("error out"=w300:errorcluster)  [unwired: 9 in]
        n106 = call "disable.vi"("error in (no error)"=w300, "Array"=w309) -> ("error out"=w311:errorcluster)  [unwired: 9 in]
        n107 = call "disable.vi"("error in (no error)"=w311, "Array"=w308) -> ("error out"=w299:errorcluster)  [unwired: 9 in]
        n108 = call "disable.vi"("error in (no error)"=w299, "Array"=w298) -> ("error out"=w294:errorcluster)  [unwired: 9 in]
        n109 = Unbundle By Name(w293) -> ("DAQ task"=w295:refnum<k21>)
        n110 = call-poly <vilib>:"DAQmx Write.vi"("task/channels in"=w295, "auto start"=TRUE, "data"=w291, "error in"=w294) -> ("task out"=w296:refnum<k21>, "error out"=w290:errorcluster)  [unwired: 9 in, 1 out]
        n111 = Bundle By Name(cluster=w293, "DAQ task"=w296) -> (w292:T1)
        n112 = case shown="False" w305 {
          tunnel: [w316 w322] -> w304
          tunnel: w303 -> [w319 w324]
          tunnel: w290 -> [w314 w320]
          frame False {
            n113 = Or(x=w314, y=w319) -> (x .or. y?=w317:bool)
            n114 = Wait (ms)(milliseconds to wait=u32 1000) -> ()  [unwired: 1 out]
            n115 = call "error_check_shutdown_freq_sweep_agilent.vi"(8:State."Measuring ref", "Boolean"=w317) -> (3:w316:T3)  [unwired: 9 in]
          }
          frame True {
            n116 = Or(x=w320, y=w324) -> (x .or. y?=w323:bool)
            n117 = call "error_check_shutdown_freq_sweep_agilent.vi"(8:State."Sweeping down", "Boolean"=w323) -> (3:w322:T3)  [unwired: 9 in]
          }
        }
      }
      frame "Measuring ref" {
        w343 = 1 ("Channel (1)")
        w344 = 0 items=["FDATA", "RDATA", "SDATA", "FMEM", "SMEM", "SDIV"] ("Data Type (0: FDATA)")
        n118 = control-ref of="Status"() -> (w357:refnum<vi>)
        n119 = Subtract(x=w333, y=w332) -> (x-y=w336:dbl)
        n120 = Subtract(x=w331, y=1.0) -> (x-y=w335:dbl)
        n121 = Divide(x=w336, y=w335) -> (x/y=w334:dbl)
        n122 = call "change_status.vi"("error in (no error)"=w356, "String"="Measuring the reference signal...", "String in"=w357) -> ("error out"=w360:errorcluster)  [unwired: 8 in]
        n123 = call "enable.vi"("error in (no error)"=w360, "Array"=w363) -> ("error out"=w352:errorcluster)  [unwired: 9 in]
        n124 = for {
          N: w331 -> [_]
          tunnel: w332 -> [w365]
          tunnel: w334 -> [w368]
          tunnel: [w364] -> w328 mode=indexing
          i -> [w367]
          n125 = Multiply(x=w368, y=w367) -> (x*y=w366:dbl)
          n126 = Add(x=w365, y=w366) -> (x+y=w364:dbl)
        }
        n127 = call "disable.vi"("error in (no error)"=w352, "Array"=w362) -> ("error out"=w359:errorcluster)  [unwired: 9 in]
        n128 = call "disable.vi"("error in (no error)"=w359, "Array"=w361) -> ("error out"=w351:errorcluster)  [unwired: 9 in]
        n129 = call "disable.vi"("error in (no error)"=w351, "Array"=w350) -> ("error out"=w339:errorcluster)  [unwired: 9 in]
        n130 = Unbundle By Name(w341) -> ("VNA name"=w342:refnum<visa-resource-name>)
        n131 = call <instrlib>:"Send Immediate Trigger.vi"("error in (no error)"=w339, "Channel (1)"=w343, "VISA resource name"=w342) -> ("error out"=w348:errorcluster, "VISA resource name out"=w349:refnum<visa-resource-name>)  [unwired: 7 in]
        n132 = while {
          shift-right: [w375] -> w347
          shift-left: w348 -> [w376]
          shift-right: [w373] -> w346
          shift-left: w349 -> [w374]
          tunnel: w325 -> [w369]
          stop <- w371 stop-if-true
          n133 = call <instrlib>:"Query Sweep Complete.vi"("error in (no error)"=w376, "VISA resource name"=w374) -> ("error out"=w375:errorcluster, "Sweep Complete"=w370:bool, "VISA resource name out"=w373:refnum<visa-resource-name>)  [unwired: 7 in]
          n134 = Or(x=w370, y=w369) -> (x .or. y?=w371:bool)
          n135 = Wait (ms)(milliseconds to wait=u32 1) -> ()  [unwired: 1 out]
        }
        n136 = call <instrlib>:"Read Data.vi"("error in (no error)"=w347, "Data Type (0: FDATA)"=w344, "Channel (1)"=w343, "VISA resource name"=w346) -> ("error out"=w338:errorcluster, "Data"=w329:dbl[], "VISA resource name out"=w345:refnum<visa-resource-name>)  [unwired: 5 in]
        n137 = Bundle By Name(cluster=w341, "VNA name"=w345) -> (w340:T1)
        n138 = Bundle By Name(cluster=w330, "Ref signal"=w329, "Frequency"=w328) -> (w327:T2)
        n139 = case shown="False" w325 {
          tunnel: [w378 w384] -> w354
          tunnel: w355 -> [w381 w386]
          tunnel: w338 -> [w377 w382]
          frame False {
            n140 = Or(x=w377, y=w381) -> (x .or. y?=w380:bool)
            n141 = call "error_check_shutdown_freq_sweep_agilent.vi"(8:State."Sweeping to H", "Boolean"=w380) -> (3:w378:T3)  [unwired: 9 in]
          }
          frame True {
            n142 = Or(x=w382, y=w386) -> (x .or. y?=w385:bool)
            n143 = call "error_check_shutdown_freq_sweep_agilent.vi"(8:State."Sweeping down", "Boolean"=w385) -> (3:w384:T3)  [unwired: 9 in]
          }
        }
      }
      frame "Sweeping to H" {
        n144 = call "field_to_voltage_convert.vi"("Start H Field (Oe)"=w404) -> ("Numeric"=w391:dbl)
        n145 = control-ref of="Status"() -> (w407:refnum<vi>)
        n146 = call "change_status.vi"("error in (no error)"=w406, "String"="Sweeping to H field...", "String in"=w407) -> ("error out"=w412:errorcluster)  [unwired: 8 in]
        n147 = call "enable.vi"("error in (no error)"=w412, "Array"=w411) -> ("error out"=w400:errorcluster)  [unwired: 9 in]
        n148 = call "disable.vi"("error in (no error)"=w400, "Array"=w409) -> ("error out"=w413:errorcluster)  [unwired: 9 in]
        n149 = call "disable.vi"("error in (no error)"=w413, "Array"=w408) -> ("error out"=w399:errorcluster)  [unwired: 9 in]
        n150 = call "disable.vi"("error in (no error)"=w399, "Array"=w398) -> ("error out"=w395:errorcluster)  [unwired: 9 in]
        n151 = Unbundle By Name(w393) -> ("DAQ task"=w394:refnum<k21>)
        n152 = call-poly <vilib>:"DAQmx Write.vi"("task/channels in"=w394, "auto start"=TRUE, "data"=w391, "error in"=w395) -> ("task out"=w396:refnum<k21>, "error out"=w390:errorcluster)  [unwired: 9 in, 1 out]
        n153 = Bundle By Name(cluster=w393, "DAQ task"=w396) -> (w392:T1)
        n154 = case shown="False" w403 {
          tunnel: [w426 w432] -> w401
          tunnel: w402 -> [w429 w434]
          tunnel: w390 -> [w424 w430]
          frame False {
            n155 = Or(x=w424, y=w429) -> (x .or. y?=w428:bool)
            n156 = Wait (ms)(milliseconds to wait=u32 1000) -> ()  [unwired: 1 out]
            n157 = call "error_check_shutdown_freq_sweep_agilent.vi"(8:State."Measuring H", "Boolean"=w428) -> (3:w426:T3)  [unwired: 9 in]
          }
          frame True {
            n158 = Or(x=w430, y=w434) -> (x .or. y?=w433:bool)
            n159 = call "error_check_shutdown_freq_sweep_agilent.vi"(8:State."Sweeping down", "Boolean"=w433) -> (3:w432:T3)  [unwired: 9 in]
          }
        }
        n160 = case shown="False" w387 {
          tunnel: w388 -> [w417 w423]
          tunnel: [w414 w418] -> w389
          frame False {
            n161 = Unbundle By Name(w417) -> ("Frequency"=w416:dbl[], "Signal"=w415:dbl[])
            n162 = Bundle("Frequency"=w416, "Signal"=w415) -> (w414:cluster{"Frequency":dbl[], "Signal":dbl[]})  [unwired: 1 in]
          }
          frame True {
            n163 = Unbundle By Name(w423) -> ("Frequency"=w420:dbl[], "Ref signal"=w422:dbl[], "Signal"=w421:dbl[])
            n164 = Subtract(x=w422, y=w421) -> (x-y=w419:dbl[])
            n165 = Bundle("Frequency"=w420, w419) -> (w418:cluster{"Frequency":dbl[], dbl[]})  [unwired: 1 in]
          }
        }
      }
      frame "Measuring H" {
        w457 = 1 ("Channel (1)")
        w458 = 0 items=["FDATA", "RDATA", "SDATA", "FMEM", "SMEM", "SDIV"] ("Data Type (0: FDATA)")
        n166 = control-ref of="Status"() -> (w469:refnum<vi>)
        n167 = Subtract(x=w446, y=w441) -> (x-y=w444:dbl)
        n168 = Subtract(x=w442, y=1.0) -> (x-y=w443:dbl)
        n169 = Divide(x=w444, y=w443) -> (x/y=w440:dbl)
        n170 = call "change_status.vi"("error in (no error)"=w470, "String"="Measuring...", "String in"=w469) -> ("error out"=w476:errorcluster)  [unwired: 8 in]
        n171 = for {
          N: w442 -> [_]
          tunnel: w441 -> [w488]
          tunnel: w440 -> [w491]
          tunnel: [w487] -> w439 mode=indexing
          i -> [w490]
          n172 = Multiply(x=w491, y=w490) -> (x*y=w489:dbl)
          n173 = Add(x=w488, y=w489) -> (x+y=w487:dbl)
        }
        n174 = call "enable.vi"("error in (no error)"=w476, "Array"=w473) -> ("error out"=w466:errorcluster)  [unwired: 9 in]
        n175 = call "disable.vi"("error in (no error)"=w466, "Array"=w472) -> ("error out"=w475:errorcluster)  [unwired: 9 in]
        n176 = call "disable.vi"("error in (no error)"=w475, "Array"=w471) -> ("error out"=w464:errorcluster)  [unwired: 9 in]
        n177 = call "disable.vi"("error in (no error)"=w464, "Array"=w465) -> ("error out"=w455:errorcluster)  [unwired: 9 in]
        n178 = Unbundle By Name(w454) -> ("VNA name"=w456:refnum<visa-resource-name>)
        n179 = call <instrlib>:"Send Immediate Trigger.vi"("error in (no error)"=w455, "Channel (1)"=w457, "VISA resource name"=w456) -> ("error out"=w462:errorcluster, "VISA resource name out"=w463:refnum<visa-resource-name>)  [unwired: 7 in]
        n180 = while {
          shift-right: [w498] -> w461
          shift-left: w462 -> [w499]
          shift-right: [w496] -> w460
          shift-left: w463 -> [w497]
          tunnel: w435 -> [w492]
          stop <- w494 stop-if-true
          n181 = call <instrlib>:"Query Sweep Complete.vi"("error in (no error)"=w499, "VISA resource name"=w497) -> ("error out"=w498:errorcluster, "Sweep Complete"=w493:bool, "VISA resource name out"=w496:refnum<visa-resource-name>)  [unwired: 7 in]
          n182 = Or(x=w493, y=w492) -> (x .or. y?=w494:bool)
          n183 = Wait (ms)(milliseconds to wait=u32 1) -> ()  [unwired: 1 out]
        }
        n184 = call <instrlib>:"Read Data.vi"("error in (no error)"=w461, "Data Type (0: FDATA)"=w458, "Channel (1)"=w457, "VISA resource name"=w460) -> ("error out"=w449:errorcluster, "Data"=w447:dbl[], "VISA resource name out"=w459:refnum<visa-resource-name>)  [unwired: 5 in]
        n185 = Bundle By Name(cluster=w454, "VNA name"=w459) -> (w453:T1)
        n186 = Bundle By Name(cluster=w448, "Signal"=w447, "Frequency"=w439) -> (w437:T2)
        n187 = case shown="True" w438 {
          tunnel: w437 -> [w480 w486]
          tunnel: [w477 w481] -> w436
          frame False {
            n188 = Unbundle By Name(w480) -> ("Frequency"=w479:dbl[], "Signal"=w478:dbl[])
            n189 = Bundle("Frequency"=w479, "Signal"=w478) -> (w477:cluster{"Frequency":dbl[], "Signal":dbl[]})  [unwired: 1 in]
          }
          frame True {
            n190 = Unbundle By Name(w486) -> ("Frequency"=w483:dbl[], "Ref signal"=w485:dbl[], "Signal"=w484:dbl[])
            n191 = Subtract(x=w485, y=w484) -> (x-y=w482:dbl[])
            n192 = Bundle("Frequency"=w483, w482) -> (w481:cluster{"Frequency":dbl[], dbl[]})  [unwired: 1 in]
          }
        }
        n193 = Or(x=w449, y=w468) -> (x .or. y?=w452:bool)
        n194 = call "error_check_shutdown_freq_sweep_agilent.vi"(8:State."Sweeping down", "Boolean"=w452) -> (3:w450:T3)  [unwired: 9 in]
      }
      frame "Sweeping down" {
        n195 = control-ref of="Status"() -> (w521:refnum<vi>)
        n196 = call "change_status.vi"("error in (no error)"=w528, "String"="Sweeping down the H field to zero...", "String in"=w521) -> ("error out"=w530:errorcluster)  [unwired: 8 in]
        n197 = call "disable.vi"("error in (no error)"=w530, "Array"=w525) -> ("error out"=w518:errorcluster)  [unwired: 9 in]
        n198 = call "disable.vi"("error in (no error)"=w518, "Array"=w526) -> ("error out"=w529:errorcluster)  [unwired: 9 in]
        n199 = call "disable.vi"("error in (no error)"=w529, "Array"=w527) -> ("error out"=w517:errorcluster)  [unwired: 9 in]
        n200 = call "disable.vi"("error in (no error)"=w517, "Array"=w516) -> ("error out"=w507:errorcluster)  [unwired: 9 in]
        n201 = Unbundle By Name(w506) -> ("VNA name"=w508:refnum<visa-resource-name>)
        n202 = call <instrlib>:"Abort Sweep.vi"("error in (no error)"=w507, "VISA resource name"=w508) -> ("error out"=w510:errorcluster, "VISA resource name out"=w511:refnum<visa-resource-name>)  [unwired: 8 in]
        n203 = Bundle By Name(cluster=w506, "VNA name"=w511) -> (w505:T1)
        n204 = Unbundle By Name(w505) -> ("DAQ task"=w509:refnum<k21>)
        n205 = call-poly <vilib>:"DAQmx Write.vi"("task/channels in"=w509, "data"=0.0, "error in"=w510) -> ("task out"=w514:refnum<k21>, "error out"=w513:errorcluster)  [unwired: 10 in, 1 out]
        n206 = call <vilib>:"DAQmx Stop Task.vi"("task/channels in"=w514, "error in"=w513) -> ("task out"=w512:refnum<k21>, "error out"=w503:errorcluster)  [unwired: 12 in]
        n207 = Bundle By Name(cluster=w505, "DAQ task"=w512) -> (w504:T1)
        n208 = case shown="False" w500 {
          tunnel: w501 -> [w535 w541]
          tunnel: [w532 w536] -> w502
          frame False {
            n209 = Unbundle By Name(w535) -> ("Frequency"=w534:dbl[], "Signal"=w533:dbl[])
            n210 = Bundle("Frequency"=w534, "Signal"=w533) -> (w532:cluster{"Frequency":dbl[], "Signal":dbl[]})  [unwired: 1 in]
          }
          frame True {
            n211 = Unbundle By Name(w541) -> ("Frequency"=w538:dbl[], "Ref signal"=w540:dbl[], "Signal"=w539:dbl[])
            n212 = Subtract(x=w540, y=w539) -> (x-y=w537:dbl[])
            n213 = Bundle("Frequency"=w538, w537) -> (w536:cluster{"Frequency":dbl[], dbl[]})  [unwired: 1 in]
          }
        }
        n214 = Or(x=w503, y=w523) -> (x .or. y?=w524:bool)
        n215 = call "error_check_shutdown_freq_sweep_agilent.vi"(8:State."Idle", "Boolean"=w524) -> (3:w522:T3)  [unwired: 9 in]
      }
      frame "Shutdown" {
        w561 = T4 3 items=["no dialog", "OK message", "continue or stop message", "OK message + warnings", "continue/stop + warnings"] ("type of dialog (OK msg:1)")
        n216 = control-ref of="Status"() -> (w572:refnum<vi>)
        n217 = call "change_status.vi"("error in (no error)"=w571, "String"="Shutting down...Sweeping field to zero...", "String in"=w572) -> ("error out"=w577:errorcluster)  [unwired: 8 in]
        n218 = call "disable.vi"("error in (no error)"=w577, "Array"=w575) -> ("error out"=w567:errorcluster)  [unwired: 9 in]
        n219 = call "disable.vi"("error in (no error)"=w567, "Array"=w574) -> ("error out"=w578:errorcluster)  [unwired: 9 in]
        n220 = Wait (ms)(milliseconds to wait=u32 1000) -> ()  [unwired: 1 out]
        n221 = call "disable.vi"("error in (no error)"=w578, "Array"=w573) -> ("error out"=w566:errorcluster)  [unwired: 9 in]
        n222 = call "disable.vi"("error in (no error)"=w566, "Array"=w565) -> ("error out"=w547:errorcluster)  [unwired: 9 in]
        n223 = Unbundle By Name(w544) -> ("DAQ task"=w546:refnum<k21>)
        n224 = call-poly <vilib>:"DAQmx Write.vi"("task/channels in"=w546, "data"=0.0, "error in"=w547) -> ("task out"=w552:refnum<k21>, "error out"=w553:errorcluster)  [unwired: 10 in, 1 out]
        n225 = call <vilib>:"DAQmx Stop Task.vi"("task/channels in"=w552, "error in"=w553) -> ("task out"=w555:refnum<k21>, "error out"=w556:errorcluster)  [unwired: 12 in]
        n226 = call <vilib>:"DAQmx Clear Task.vi"("task in"=w555, "error in"=w556) -> ("error out"=w549:errorcluster)  [unwired: 13 in]
        n227 = Unbundle By Name(w544) -> ("VNA name"=w545:refnum<visa-resource-name>)
        n228 = call <instrlib>:"Abort Sweep.vi"("error in (no error)"=w549, "VISA resource name"=w545) -> ("error out"=w551:errorcluster, "VISA resource name out"=w550:refnum<visa-resource-name>)  [unwired: 8 in]
        n229 = call <instrlib>:"Close.vi"("error in (no error)"=w551, "VISA resource name"=w550) -> ("error out"=w548:errorcluster)  [unwired: 9 in]
        n230 = Unbundle By Name(w544) -> ("Gaussmeter Name"=w543:refnum<visa-resource-name>)
        n231 = call <instrlib>:"LSCI 475 Close.vi"("VISA session"=w543, "error in (no error)"=w548) -> ("error out"=w542:errorcluster)  [unwired: 13 in]
        n232 = property on="SpectrumGraph" class="XYGraph (strict)"(error in=w542, "Value"=cluster{"Field":dbl[], "Signal":dbl[]} {"Field"=[], "Signal"=[]} ("SpectrumGraph")) -> (error out=w559:errorcluster)  [unwired: 1 in, 1 out]
        n233 = control-ref of="Status"() -> (w564:refnum<vi>)
        n234 = call "change_status.vi"("error in (no error)"=w559, "String"="Off", "String in"=w564) -> ("error out"=w562:errorcluster)  [unwired: 8 in]
        n235 = call <vilib>:"Simple Error Handler.vi"("type of dialog (OK msg:1)"=w561, "error in (no error)"=w562) -> ("error out"=w560:errorcluster)  [unwired: 3 in, 4 out]
      }
    }
    "SpectrumGraph" <- w48
    n236 = Unbundle By Name(w42) -> ("Gaussmeter Name"=w45:refnum<visa-resource-name>)
    n237 = call <instrlib>:"LSCI 475 Data Field.vi"("error in (no error)"=w46, "VISA session"=w45) -> ("error out"=w44:errorcluster, "Field Reading"=→"Field, Oe":dbl, "dup VISA session"=w43:refnum<visa-resource-name>)  [unwired: 7 in]
    n238 = event shown="[1] \"SpectrumGraph\": Mouse Down" {
      selector: _ -> [_ _ _]
      dyn-events: _ -> [_ _ _]
      timeout: 1 -> [_ _ _]
      tunnel: w47 -> [_ _ w90]
      event Timeout {
        n239 = event-data() -> ()  [unwired: 1 in, 3 out]
      }
      event "SpectrumGraph": Mouse Down {
        n240 = event-data() -> ("CtlRef"=w77:refnum<vi>, "Coords"=w78:T5)  [unwired: 1 in]
        n241 = invoke on="Invoke Node" class="XYGraph (strict)" method="Map Coords To XY"(reference=w77, "Coords"=w78) -> ("Map Coords To XY"=w79:bool, "XY"=w80:cluster{"X":dbl, "Y":dbl})  [unwired: 5 in, 5 out]
        n242 = case shown="True" w79 {
          tunnel: w80 -> [_ w81]
          frame False {
          }
          frame True {
            n243 = property on="Cursor" class="Clust (strict)"("Value"=w81) -> ()  [unwired: 2 in, 2 out]
          }
        }
      }
      event "Save Button": Value Change {
        n244 = event-data() -> ()  [unwired: 1 in, 1 out]
        n245 = Unbundle By Name(w90) -> ("Ref signal"=w89:dbl[], "Frequency"=w86:dbl[], "Ref signal"=w85:dbl[], "Signal"=w84:dbl[])
        n246 = Array Size(array=w89) -> (size(s)=w88:i32)
        n247 = Equal To 0?(x=w88) -> (x = 0?=w87:bool)
        n248 = case shown="False" w87 {
          tunnel: w86 -> [w94 w99]
          tunnel: w85 -> [w96 _]
          tunnel: w84 -> [w95 w98]
          tunnel: [w94 w99] -> w83
          tunnel: [w97 w98] -> w82
          frame False {
            n249 = Subtract(x=w96, y=w95) -> (x-y=w97:dbl[])
          }
          frame True {
          }
        }
        n250 = call "Convert to Dynamic Data"("Array"=w83) -> ("Dynamic Data Type"=w93:dynamicdata)  [unwired: 3 in]
        n251 = call "Convert to Dynamic Data2"("Array"=w82) -> ("Dynamic Data Type"=w91:dynamicdata)  [unwired: 3 in]
        n252 = Merge Signals(w93, w91) -> (w92:dynamicdata)
        n253 = call "Write To Measurement File"("Signals"=w92) -> ()  [unwired: 16 in, 3 out]
      }
    }
    n254 = Bundle By Name(cluster=w42, "Gaussmeter Name"=w43) -> (w41:T1)
  }
  "Error Out" <- w25
